vi "Trajectory.vi"(6 "HomeXY(pixels)":cluster{dbl, dbl}, 7 "PixelmmRatio":dbl format="%#_13g", 8 "Horizontal Edges":T2(array[cluster]) {"Point2 (Real-World)"."Y" format="%.2f"; "Point2 (Real-World)"."X" format="%.2f"; "Point1 (Real-World)"."Y" format="%.2f"; "Point1 (Real-World)"."X" format="%.2f"; "Point2 (Pixels)"."Y" format="%.2f"; "Point2 (Pixels)"."X" format="%.2f"; "Point1 (Pixels)"."Y" format="%.2f"; "Point1 (Pixels)"."X" format="%.2f"}, 9 "Vertical Edges":T2(array[cluster]) {"Point2 (Real-World)"."Y" format="%.2f"; "Point2 (Real-World)"."X" format="%.2f"; "Point1 (Real-World)"."Y" format="%.2f"; "Point1 (Real-World)"."X" format="%.2f"; "Point2 (Pixels)"."Y" format="%.2f"; "Point2 (Pixels)"."X" format="%.2f"; "Point1 (Pixels)"."Y" format="%.2f"; "Point1 (Pixels)"."X" format="%.2f"}, 10 "Puck":T3(array[cluster]) {"Position"."Y" format="%.2f"; "Position"."X" format="%.2f"}, 11 "Players":T3(array[cluster]) {"Position"."Y" format="%.2f"; "Position"."X" format="%.2f"}) -> (0 "Kicker XY":cluster{dbl, dbl}, 1 "ChosenEnergy":dbl, 2 "ChosenPathIdx":i32, 3 "TrajectoryArray":T1, 4 "Angle":dbl, 5 "PuckCentre":cluster{"PuckX":sgl, "PuckY":sgl})   [LabVIEW 2017]
uses:
  <vilib>/imath/engines/lvmath2/RunTimeEngine/IndexReplace/NIMS V(S)=S.vi
  <instcachedir>/0/NIMS V(S)=S_EDDEB2B900FD4B108B325BCE58B17C3D.lvgen/NIMS V(S)=S_EDDEB2B900FD4B108B325BCE58B17C3D_000.vi
  <vilib>/imathl/engines/lvmath/Functions/Error Handling/Create Error.vi
  <vilib>/imath/engines/lvmath2/RunTimeEngine/IndexRead/NIMS V(S).vi
  <instcachedir>/0/NIMS V(S)_0488751826AF41519A22953C041130DC.lvgen/NIMS V(S)_0488751826AF41519A22953C041130DC_000.vi
  <instcachedir>/0/NIMS V(S)_0488751826AF41519A22953C041130DC.lvgen/NIMS V(S)_0488751826AF41519A22953C041130DC_004.vi
  <vilib>/imath/engines/lvmath2/RunTimeEngine/ErrorHandling/NIMS_Create Error From Enums.vi
  <instcachedir>/0/NIMS V(S)=S_EDDEB2B900FD4B108B325BCE58B17C3D.lvgen/NIMS V(S)=S_EDDEB2B900FD4B108B325BCE58B17C3D_004.vi
  <instcachedir>/0/NIMS V(S)=S_EDDEB2B900FD4B108B325BCE58B17C3D.lvgen/NIMS V(S)=S_EDDEB2B900FD4B108B325BCE58B17C3D_003.vi
  <vilib>/imath/engines/lvmath2/RunTimeEngine/BuiltInFunctions/cos/NIMS_cos(C).vi
  <instcachedir>/0/NIMS_cos(C)_AA2BCF4E9A6E496BB2D8610C99CE3BDF.lvgen/NIMS_cos(C)_AA2BCF4E9A6E496BB2D8610C99CE3BDF_001.vi
  <instcachedir>/0/NIMS V(S)=S_EDDEB2B900FD4B108B325BCE58B17C3D.lvgen/NIMS V(S)=S_EDDEB2B900FD4B108B325BCE58B17C3D_001.vi
  <instcachedir>/0/NIMS V(S)_0488751826AF41519A22953C041130DC.lvgen/NIMS V(S)_0488751826AF41519A22953C041130DC_003.vi
  <vilib>/imath/engines/lvmath2/RunTimeEngine/BuiltInFunctions/sin/NIMS_sin(C).vi
  <instcachedir>/0/NIMS_sin(C)_6D39E71311DB42CFBE2ED5287D1CD3DE.lvgen/NIMS_sin(C)_6D39E71311DB42CFBE2ED5287D1CD3DE_001.vi
  <vilib>/imath/engines/lvmath2/RunTimeEngine/RangeToken/NIMS_Range_R3 - Integer.vi
  <instcachedir>/0/NIMS_Range_R3 - Integer_5F780326EA7B4D7DA3CAB5327CCF1FD4.lvgen/NIMS_Range_R3 - Integer_5F780326EA7B4D7DA3CAB5327CCF1FD4_000.vi
  <vilib>/imath/engines/lvmath2/RunTimeEngine/CommandStatement/MC_CommandStatement_break.vi
  <vilib>/imath/engines/lvmath2/RunTimeEngine/BuiltInFunctions/abs/NIMS_abs(signed).vi
  <instcachedir>/0/NIMS_abs(signed)_C4FCB8E6058B49B797C7C8D53CA5F6EC.lvgen/NIMS_abs(signed)_C4FCB8E6058B49B797C7C8D53CA5F6EC_002.vi
  <vilib>/imath/engines/lvmath/Functions/Error Handling/MergeErrorsWrapper.vi
  <vilib>/imath/engines/lvmath2/RunTimeEngine/BuiltInFunctions/tan/NIMS_tan(C).vi
  <instcachedir>/0/NIMS_tan(C)_6BC19E5424E24807BE8B7BD5A8682FBF.lvgen/NIMS_tan(C)_6BC19E5424E24807BE8B7BD5A8682FBF_001.vi
  <vilib>/imath/engines/lvmath2/RunTimeEngine/ArithmeticOperatorToken/NIMS_ArithmeticOperator_power(S).vi
  <instcachedir>/0/NIMS_ArithmeticOperator_power(S)_6724F8489F734D67A0FA3662C6F9A073.lvgen/NIMS_ArithmeticOperator_power(S)_6724F8489F734D67A0FA3662C6F9A073_010.vi
  <vilib>/imath/engines/lvmath2/RunTimeEngine/NodeEndStatement/NIMS_NodeEndStatement_Output.vi
  <instcachedir>/0/NIMS_NodeEndStatement_Output_53EC0D466D134D7ABD903AC30B43404B.lvgen/NIMS_NodeEndStatement_Output_53EC0D466D134D7ABD903AC30B43404B_008.vi
  <instcachedir>/0/NIMS_NodeEndStatement_Output_53EC0D466D134D7ABD903AC30B43404B.lvgen/NIMS_NodeEndStatement_Output_53EC0D466D134D7ABD903AC30B43404B_009.vi
  <vilib>/imath/engines/lvmath2/RunTimeEngine/ErrorHandling/NIMS_Finalize Error.vi
panel:
  out "Lg":dbl[](array[numeric])
  out "Lw Left":dbl[](array[numeric])
  out "Lw right":dbl[](array[numeric])
  out "Puck":sgl[](array[numeric])
  out "isPossible 2":i32[](array[numeric])
  out "energy":dbl[](array[numeric])
  out "Ptwy":dbl
  out "Ptwx":dbl
  out "Ptfy":cdb
  out "Ptfx":cdb
  out "playerPoints":dbl[](array[numeric])
  out "energyRes":dbl
  out "isPossible":i32
  out "DorR":i32
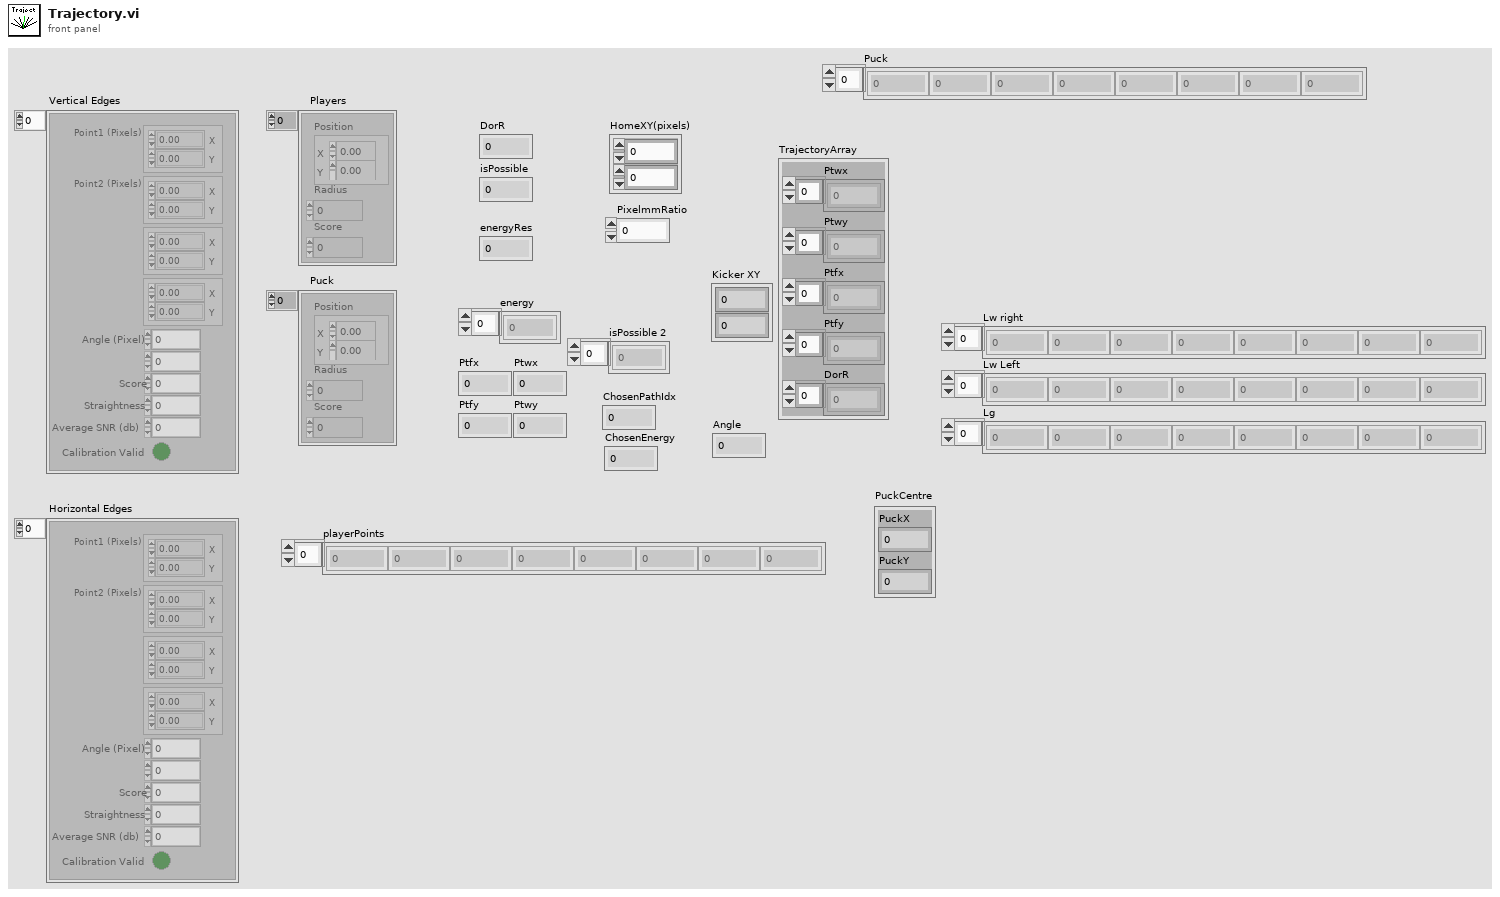
[diagram p1: front panel]
types:
  T1 = cluster{"Ptwx":dbl[], "Ptwy":dbl[], "Ptfx":dbl[], "Ptfy":dbl[], "DorR":i32[]}
  T2 = cluster{"Point1 (Pixels)":cluster{"X":sgl, "Y":sgl}, "Point2 (Pixels)":cluster{"X":sgl, "Y":sgl}, "Point1 (Real-World)":cluster{"X":sgl, "Y":sgl}, "Point2 (Real-World)":cluster{"X":sgl, "Y":sgl}, "Angle (Pixel)":dbl, "Angle (Real-World)":dbl, "Score":dbl, "Straightness":dbl, "Average SNR (db)":dbl, "Calibration Valid":bool}[]
  T3 = cluster{"Position":cluster{"X":sgl, "Y":sgl}, "Radius":dbl, "Score":dbl}[]
  T4 = cluster{"Puck[0]":cluster{"Position":cluster{"X":sgl, "Y":sgl}, "Radius":dbl, "Score":dbl}, "Puck[1]":cluster{"Position":cluster{"X":sgl, "Y":sgl}, "Radius":dbl, "Score":dbl}, "Puck[2]":cluster{"Position":cluster{"X":sgl, "Y":sgl}, "Radius":dbl, "Score":dbl}, "Puck[3]":cluster{"Position":cluster{"X":sgl, "Y":sgl}, "Radius":dbl, "Score":dbl}, "Puck[4]":cluster{"Position":cluster{"X":sgl, "Y":sgl}, "Radius":dbl, "Score":dbl}, "Puck[5]":cluster{"Position":cluster{"X":sgl, "Y":sgl}, "Radius":dbl, "Score":dbl}, "Puck[6]":cluster{"Position":cluster{"X":sgl, "Y":sgl}, "Radius":dbl, "Score":dbl}, "Puck[7]":cluster{"Position":cluster{"X":sgl, "Y":sgl}, "Radius":dbl, "Score":dbl}, "Puck[8]":cluster{"Position":cluster{"X":sgl, "Y":sgl}, "Radius":dbl, "Score":dbl}}
  T5 = cluster{"Position":cluster{"X":sgl, "Y":sgl}, "Radius":dbl, "Score":dbl}
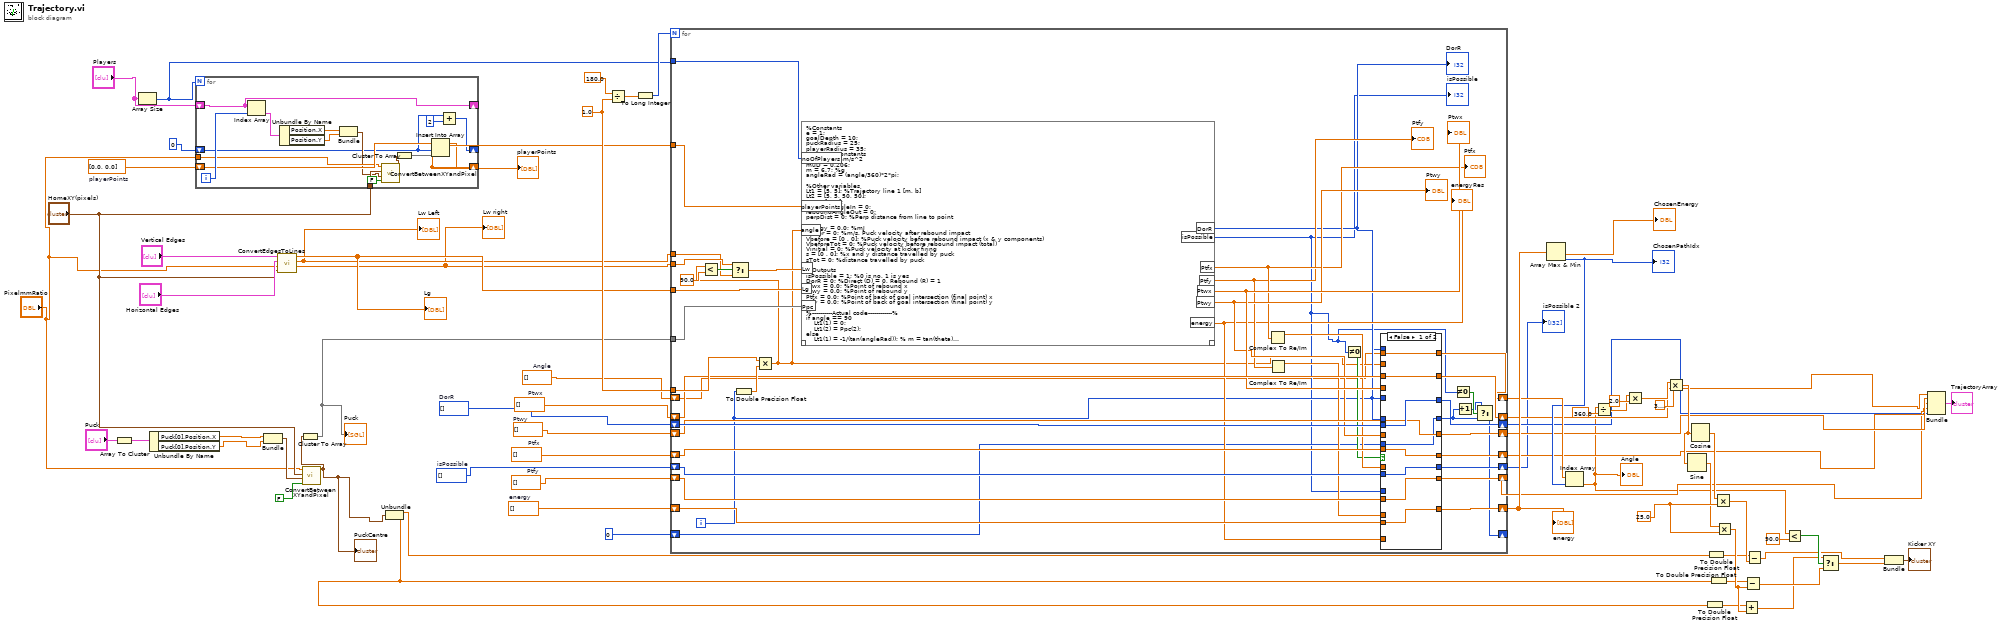
[diagram p0: block diagram]
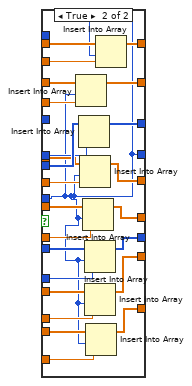
[diagram p2: hidden frame]
diagram:
  w4 = dbl[] []  # Angle
  w30 = i32[] []  # isPossible
  w29 = i32[] []  # DorR
  w31 = dbl[] []  # Ptfy
  w32 = dbl[] []  # Ptwy
  w33 = dbl[] []  # Ptwx
  w47 = 25.0
  w56 = dbl[] []  # energy
  w62 = dbl[] [0.0, 0.0]  # playerPoints
  w64 = dbl[] []  # Ptfx
  w65 = 1.0
  n1 = Array To Cluster(array="Puck") -> (cluster=w59:T4)
  n2 = Array Size(array="Players") -> (size(s)=w34:i32)
  n3 = Unbundle By Name(w59) -> ("Puck[0].Position.X"=w10:sgl, "Puck[0].Position.Y"=w8:sgl)
  n4 = for {
    N: w34 -> [_]
    shift-right: [w80] -> _
    shift-left: "Players" -> [w80]
    shift-right: [w81] -> w61
    shift-left: w62 -> [w82]
    tunnel: "HomeXY(pixels)" -> [w78]
    tunnel: "PixelmmRatio" -> [w76]
    shift-right: [w69] -> _
    shift-left: 0 -> [w71]
    i -> [w83]
    n5 = Index Array(array=w80, index=w83) -> (element=w84:T5)
    n6 = Unbundle By Name(w84) -> ("Position.X"=w75:sgl, "Position.Y"=w74:sgl)
    n7 = Bundle("X"=w75, "Y"=w74) -> (w73:cluster{"X":sgl, "Y":sgl})  [unwired: 1 in]
    n8 = call "ConvertBetweenXYandPixel.vi"("XYtoPixels"=FALSE, "PointToConvert"=w73, "HomeXY(pixels)"=w78, "Pixel/mm"=w76) -> ("Point"=w77:cluster{sgl, sgl})  [unwired: 7 in]
    n9 = Cluster To Array(cluster=w77) -> (array=w79:sgl[])
    n10 = Insert Into Array(array=w82, index=w71, new element=w79) -> (w81:dbl[])
    n11 = Add(x=w71, y=2) -> (x+y=w69:i32)
  }
  "playerPoints" <- w61
  n12 = Bundle("X"=w10, "Y"=w8) -> (w19:cluster{"X":sgl, "Y":sgl})  [unwired: 1 in]
  n13 = call "ConvertEdgesToLines.vi"("HomeXY(pixels)"="HomeXY(pixels)", "PixelmmRatio"="PixelmmRatio", "Horizontal Edges"="Horizontal Edges", "Vertical Edges"="Vertical Edges") -> ("Lw Right"=w11:dbl[], "Lw Left"=w12:dbl[], "Lg"=w13:dbl[])  [unwired: 5 in]
  "Lw right" <- w11
  "Lw Left" <- w12
  "Lg" <- w13
  n14 = call "ConvertBetweenXYandPixel.vi"("XYtoPixels"=FALSE, "PointToConvert"=w19, "HomeXY(pixels)"="HomeXY(pixels)", "Pixel/mm"="PixelmmRatio") -> ("Point"=w3:cluster{sgl, sgl})  [unwired: 7 in]
  "PuckCentre" <- w3
  n15 = Cluster To Array(cluster=w3) -> (array=w14:sgl[])
  "Puck" <- w14
  n16 = Unbundle(w3) -> (w9:sgl, w7:sgl)
  n17 = Divide(x=180.0, y=w65) -> (x/y=w66:dbl)
  n18 = To Long Integer(number=w66) -> (32bit integer=w67:i32)
  n19 = for {
    N: w67 -> [_]
    tunnel: w65 -> [w127]
    shift-right: [w99] -> w24
    shift-left: w64 -> [w114]
    tunnel: w12 -> [w121]
    tunnel: w11 -> [w122]
    tunnel: w13 -> [w125]
    tunnel: w61 -> [w119]
    tunnel: w14 -> [w126]
    shift-right: [w96] -> w55
    shift-left: w56 -> [w111]
    tunnel: w34 -> [w118]
    shift-right: [w102] -> w26
    shift-left: w33 -> [w117]
    shift-right: [w101] -> w22
    shift-left: w29 -> [w116]
    shift-right: [w100] -> w25
    shift-left: w32 -> [w115]
    shift-right: [w98] -> w20
    shift-left: w30 -> [w113]
    shift-right: [w97] -> w23
    shift-left: w31 -> [w112]
    shift-right: [w94] -> w28
    shift-left: w4 -> [w85]
    shift-right: [w86] -> _
    shift-left: 0 -> [w91]
    i -> [w92]
    n20 = To Double Precision Float(number=w92) -> (double precision float=w128:dbl)
    n21 = Multiply(x=w127, y=w128) -> (x*y=w93:dbl)
    n22 = Less?(x=w93, y=90.0) -> (x < y?=w123:bool)
    n23 = Select(t=w122, s=w123, f=w121) -> (s? t:f=w120:dbl[])
    n24 = mathscript code="%Constants\ne = 1;\ngoalDepth = 10;\npuckRadius = 25;\nplayerRadius = 35;\n%Energy Constants \ng = 9.81; %m/s^2\nmuD = 0.206;\nm = 6.7; %g\nangleRad = (angle/360)*2*pi;\n\n%Other variables\nLt1 = [5, 5]; %Trajectory line 1 [m, b]\nLt2 = [5, 5, 50, 50];\nPtg = [5, 5];\nreboundAngleIn = 0;\nreboundAngleOut = 0;\nperpDist = 0; %Perp distance from line to point\n\nenergy = 0.0; %mJ\nVafter = 0; %m/s, Puck velocity after rebound impact\nVbefore = [0 , 0]; %Puck velocity before rebound impact (x & y components)\nVbeforeTot = 0; %Puck velocity before rebound impact (total)\nVinitial = 0; %Puck velocity at kicker firing\ns = [0 , 0]; %x and y distance travelled by puck\nsTot = 0; %distance travelled by puck\n\n%Outputs\nisPossible = 1; %0 is no, 1 is yes\nDorR = 0; %Direct (D) = 0, Rebound (R) = 1\nPtwx = 0.0; %Point of rebound x\nPtwy = 0.0; %Point of rebound y\nPtfx = 0.0; %Point of back of goal intersection (final point) x\nPtfy = 0.0; %Point of back of goal intersection (final point) y\n\n%----------Actual code------------%\nif angle == 90\n    Lt1(1) = 0;\n    Lt1(2) = Ppc(2);\nelse\n    Lt1(1) = -1/(tan(angleRad)); % m = tan(theta)\n    Lt1(2) = Ppc(2) - (Lt1(1)*Ppc(1)); % b = y - mx\nend\n\n%offset lines and intersection points\nif angle<90\n    Lw(2) = Lw(2) + (puckRadius/(cos(atan(Lw(1)))));\n    Lw(3) = Lw(3) - puckRadius; %y\n    Lw(4) = Lw(4) + puckRadius;\nelse\n    Lw(2) = Lw(2) - (puckRadius/(cos(atan(Lw(1)))));\n    Lw(3) = Lw(3) - puckRadius;\n    Lw(4) = Lw(4) - puckRadius;\nend\n\nif Lg(1) == 0\n    Lg(2) = Lg(2) - puckRadius;\nelse\n    Lg(2) = Lg(2) - (puckRadius/(sin(atan(Lg(1)))));\nend\nLg(3) = Lg(3) - puckRadius; \nLg(4) = Lg(4) - puckRadius; \nLg(5) = Lg(5) - puckRadius;\nLg(6) = Lg(6) + puckRadius; \n\n%-------------------Intersects with players?----------------%\nfor i = 1:2:noOfPlayers\n    if playerPoints(i) > 0\n        perpDist = ((Lt1(1)*playerPoints(i))+(-1*playerPoints(i+1))+Lt1(2))/(sqrt((Lt1(1)^2)+1));\n        if abs(perpDist) < 30 %(puckRadius+playerRadius)\n            isPossible = 0;\n        end\n    end\nend\n\nif isPossible == 1    \n    %-----------Check if intersects with goal-------------%\n    if Lg(1) == 0\n        Ptg(1) = Lg(2);\n    else\n        Ptg(1) = (Lt1(2)-Lg(2))/(Lg(1)-Lt1(1));\n    end\n    Ptg(2) = (Lt1(1)*Ptg(1))+Lt1(2);\n    if (Ptg(2) < Lg(4)) && (Ptg(2) > Lg(6))\n        if angle == 90\n            Ptfy = Ptg(2);\n        else\n            Ptfy = Ptg(2) + (goalDepth * Lt1(1));\n        end\n        Ptfx = Ptg(1) + goalDepth;\n    elseif ((angle > 90) && (Ptg(2) > Lw(4))) || ((angle < 90) && (Ptg(2) < Lw(4)))\n        DorR = 1;\n        %Check intersection with wall and calculate rebound\n        Ptwx = (Lw(2)-Lt1(2))/(Lt1(1)-Lw(1));\n        Ptwy = (Lw(1)*Ptwx) + Lw(2);\n        %Calculate rebound angle\n        reboundAngleIn = (pi/2) - angleRad;\n        reboundAngleOut = (pi/2) - (atan(e*tan(reboundAngleIn))); %90 - tan-1(e*tan(angle))\n        %Convert angle and point into line\n        Lt2(1) = -1*tan(reboundAngleOut);\n        Lt2(2) = Ptwy - (Lt2(1)*Ptwx); % b = y - mx\n        %Check intersection with goal\n        if Lg(1) == 0\n            Ptg(1) = Lg(2);\n        else\n            Ptg(1) = (Lt2(2)-Lg(2))/(Lg(1)-Lt2(1));\n        end\n        Ptg(2) = (Lt2(1)*Ptg(1))+Lt2(2);\n        if (Ptg(2) < Lg(4)) && (Ptg(2) > Lg(6))\n            if angle == 90\n                Ptfy = Ptg(2);\n            else\n                Ptfy = Ptg(2) + (goalDepth * Lt2(1));\n            end\n            Ptfx = Ptg(1) + goalDepth;\n            %-------------------Intersects with players?----------------%\n            for i = 1:2:noOfPlayers\n                if playerPoints(i) > 0\n                    perpDist = ((Lt2(1)*playerPoints(i))+(-1*playerPoints(i+1))+Lt2(2))/(sqrt((Lt2(1)^2)+1));\n                    if abs(perpDist) < 30 %(puckRadius+playerRadius)\n                        isPossible = 0;\n                    end\n                end\n            end\n        else\n            isPossible = 0;\n        end\n    else\n        isPossible = 0;\n    end\nend\n\n%need to calculate energy resolution\nif isPossible==1\n    if DorR == 0 %For direct shots\n        s(1) = (Ptfx - Ppc(1)) / 1000; %Find x distance travelled\n        s(2) = (Ptfy - Ppc(2)) / 1000; %Find y distance travelled\n        sTot = SQRT((s(1)^2)+(s(2)^2)); %Find total distance travelled\n        Vinitial = SQRT(2*muD*g*sTot); %Find puck output V required\n        energy = 0.5*m*(Vinitial^2);\n    end\n    if DorR == 1 %For rebound shots\n        s(1) = (Ptfx- Ptwx) / 1000; %Find x distance travelled rebound to final\n        s(2) = (Ptfy - Ptwy) / 1000; %Find y distance travelled rebound to final\n        sTot = SQRT((s(1)^2)+(s(2)^2)); %Find total distance travelled rebound to final\n        Vafter = SQRT(2*muD*g*sTot); %V just after rebound\n        Vbefore(1) = (Vafter * sin(reboundAngleOut)) / e; %x-Velocity component before rebound\n        Vbefore(2) = (Vafter * cos(reboundAngleOut)); %y-Velocity component before rebound\n        VbeforeTot = SQRT((Vbefore(1)^2)+(Vbefore(2)^2)); %Velocity before rebound\n        s(1) = (Ptwx - Ppc(1)) / 1000; %Find x distance travelled inital to rebound\n        s(2) = (Ptwy - Ppc(2)) / 1000; %Find y distance travelled inital to rebound\n        sTot = SQRT((s(1)^2)+(s(2)^2)); %Find total distance travelled inital to rebound\n        Vinitial = SQRT((VbeforeTot^2)+(2*muD*g*sTot)); %Find puck output V required\n        energy = 0.5*m*(Vinitial^2);\n    end\nend"("angle"=w93, "playerPoints"=w119, "Lw"=w120, "Lg"=w125, "Ppc"=w126, "noOfPlayers"=w118) -> ("isPossible"=w90:i32, "DorR"=w103:i32, "energy"=w104:cdb, "Ptfx"=w108:cdb, "Ptfy"=w107:cdb, "Ptwx"=w110:cdb, "Ptwy"=w109:cdb)  [unwired: 1 in, 1 out]
    "DorR" <- w103
    "isPossible" <- w90
    "energyRes" <- w104
    "Ptfx" <- w108
    "Ptfy" <- w107
    "Ptwx" <- w110
    "Ptwy" <- w109
    n25 = Complex To Re/Im(x + iy=w108) -> (x=w106:dbl)  [unwired: 1 out]
    n26 = Complex To Re/Im(x + iy=w107) -> (x=w105:dbl)  [unwired: 1 out]
    n27 = Not Equal To 0?(x=w90) -> (x != 0?=w95:bool)
    n28 = case shown="False" w95 {
      tunnel: w117 -> [w137 w162]
      tunnel: w116 -> [w136 w161]
      tunnel: w115 -> [w134 w160]
      tunnel: w114 -> [w133 w159]
      tunnel: w113 -> [w135 w158]
      tunnel: w112 -> [w132 w157]
      tunnel: w111 -> [w131 w156]
      tunnel: w92 -> [_ _]
      tunnel: w110 -> [_ w155]
      tunnel: w109 -> [_ w154]
      tunnel: w106 -> [_ w153]
      tunnel: w105 -> [_ w152]
      tunnel: w104 -> [_ w151]
      tunnel: w103 -> [_ w150]
      tunnel: w90 -> [_ w149]
      tunnel: [w137 w148] -> w102
      tunnel: [w136 w147] -> w101
      tunnel: [w134 w146] -> w100
      tunnel: [w133 w145] -> w99
      tunnel: [w135 w144] -> w98
      tunnel: [w132 w143] -> w97
      tunnel: [w131 w142] -> w96
      tunnel: w85 -> [w130 w141]
      tunnel: [w130 w140] -> w94
      tunnel: w93 -> [_ w139]
      tunnel: w92 -> [_ _]
      tunnel: w91 -> [w129 w138]
      tunnel: [w129 w138] -> w88
      frame False {
      }
      frame True {
        n29 = Insert Into Array(array=w162, index=w138, new element=w155) -> (w148:dbl[])
        n30 = Insert Into Array(array=w161, new element=w150) -> (w147:i32[])  [unwired: 1 in]
        n31 = Insert Into Array(array=w160, index=w138, new element=w154) -> (w146:dbl[])
        n32 = Insert Into Array(array=w159, index=w138, new element=w153) -> (w145:dbl[])
        n33 = Insert Into Array(array=w158, index=w138, new element=w149) -> (w144:i32[])
        n34 = Insert Into Array(array=w157, index=w138, new element=w152) -> (w143:dbl[])
        n35 = Insert Into Array(array=w156, index=w138, new element=w151) -> (w142:dbl[])
        n36 = Insert Into Array(array=w141, index=w138, new element=w139) -> (w140:dbl[])
      }
    }
    n37 = Not Equal To 0?(x=w90) -> (x != 0?=w89:bool)
    n38 = Increment(x=w88) -> (x+1=w87:i32)
    n39 = Select(t=w87, s=w89, f=w88) -> (s? t:f=w86:i32)
  }
  "energy" <- w55
  "isPossible 2" <- w20
  n40 = Array Max & Min(array=w55) -> (min value=→"ChosenEnergy":dbl, min index (indices)=w27:i32)  [unwired: 2 out]
  "ChosenPathIdx" <- w27
  n41 = Index Array(array=w28, index=w27) -> (element=w5:dbl)
  "Angle" <- w5
  n42 = Divide(x=w5, y=360.0) -> (x/y=w51:dbl)
  n43 = Multiply(x=w51, y=2.0) -> (x*y=w50:dbl)
  n44 = Multiply(x=w50, y=3.141592653589793) -> (x*y=w48:dbl)
  n45 = Sine(x=w48) -> (sin(x)=w45:dbl)
  n46 = Cosine(x=w48) -> (cos(x)=w46:dbl)
  n47 = To Double Precision Float(number=w7) -> (double precision float=w40:dbl)
  n48 = To Double Precision Float(number=w9) -> (double precision float=w42:dbl)
  n49 = To Double Precision Float(number=w7) -> (double precision float=w41:dbl)
  n50 = Multiply(x=w46, y=w47) -> (x*y=w44:dbl)
  n51 = Multiply(x=w45, y=w47) -> (x*y=w43:dbl)
  n52 = Add(x=w40, y=w43) -> (x+y=w1:dbl)
  n53 = Subtract(x=w41, y=w43) -> (x-y=w2:dbl)
  n54 = Subtract(x=w42, y=w44) -> (x-y=w37:dbl)
  n55 = Less?(x=w5, y=90.0) -> (x < y?=w38:bool)
  n56 = Select(t=w1, s=w38, f=w2) -> (s? t:f=w36:dbl)
  n57 = Bundle(w37, w36) -> (→"Kicker XY":cluster{dbl, dbl})  [unwired: 1 in]
  n58 = Bundle("Ptwx"=w26, "Ptwy"=w25, "Ptfx"=w24, "Ptfy"=w23, "DorR"=w22) -> (→"TrajectoryArray":T1)  [unwired: 1 in]
